vi "selectByTime.vi"(0 "0-array (ch1 length)":i32[](array[numeric]), 1 "router channels":u8[](array[numeric]), 2 "macro times":i32[](array[numeric]), 3 "0-array (ch2 length)":i32[](array[numeric]), 4 "Cross Ch2 (hardware)":dbl, 5 "Cross Ch1 (hardware)":dbl) -> (6 "macro times ch2":i32[](array[numeric]), 7 "macro times ch1":i32[](array[numeric]))   [LabVIEW 2009]
panel:
  out "Numeric":i32
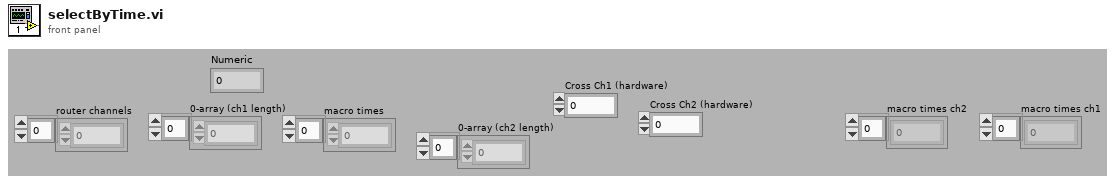
[diagram p1: front panel]
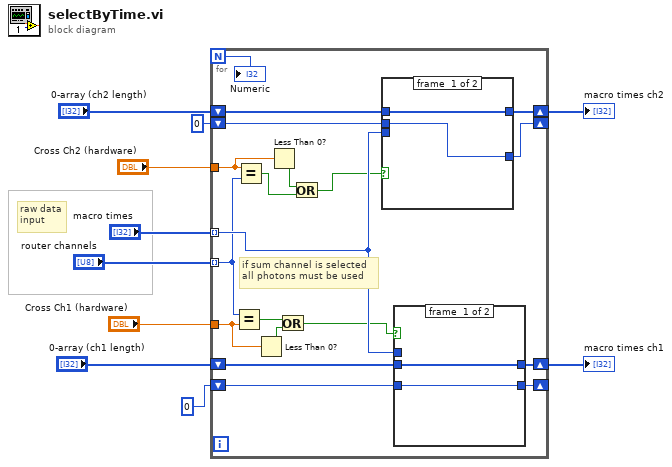
[diagram p0: block diagram]
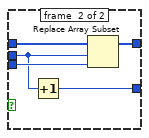
[diagram p2: hidden frame]
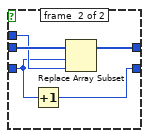
[diagram p3: hidden frame]
diagram:
  # "raw data\ninput"
  n1 = for {
    N -> [w11]
    tunnel: "macro times" -> [w21] mode=indexing
    shift-right: [w28] -> w4
    shift-left: "0-array (ch1 length)" -> [w29]
    tunnel: "Cross Ch1 (hardware)" -> [w15]
    tunnel: "router channels" -> [w18] mode=indexing
    shift-right: [w26] -> _
    shift-left: u32 0 ("element") -> [w27]
    tunnel: "Cross Ch2 (hardware)" -> [w14]
    shift-right: [w23] -> w6
    shift-left: "0-array (ch2 length)" -> [w25]
    shift-right: [w22] -> _
    shift-left: u32 0 ("element") -> [w24]
    # "if sum channel is selected\nall photons must be used"
    n2 = Equal?(x=w18, y=w15) -> (x = y?=w20:bool)
    n3 = Equal?(x=w14, y=w18) -> (x = y?=w12:bool)
    n4 = Less Than 0?(x=w15) -> (x < 0?=w16:bool)
    n5 = Less Than 0?(x=w14) -> (x < 0?=w13:bool)
    n6 = Or(x=w20, y=w16) -> (x .or. y?=w17:bool)
    n7 = Or(x=w13, y=w12) -> (x .or. y?=w19:bool)
    n8 = case shown="True" w19 {
      tunnel: w25 -> [w31 w36]
      tunnel: [w31 w35] -> w23
      tunnel: w21 -> [_ w34]
      tunnel: w24 -> [w30 w32]
      tunnel: [w30 w33] -> w22
      frame #0 {
      }
      frame #1 {
        n9 = Increment(x=w32) -> (x+1=w33:u32)
        n10 = Replace Array Subset(array=w36, new element=w34, index=w32) -> (w35:i32[])
      }
    }
    n11 = case shown="True" w17 {
      tunnel: w29 -> [w38 w43]
      tunnel: [w38 w42] -> w28
      tunnel: w21 -> [_ w41]
      tunnel: w27 -> [w37 w39]
      tunnel: [w37 w40] -> w26
      frame #0 {
      }
      frame #1 {
        n12 = Increment(x=w39) -> (x+1=w40:u32)
        n13 = Replace Array Subset(array=w43, new element=w41, index=w39) -> (w42:i32[])
      }
    }
    "Numeric" <- w11
  }
  "macro times ch2" <- w6
  "macro times ch1" <- w4
